vi "Get Index By Serial Number.vi"(8 "error in (no error)":errorcluster, 11 "Serial Number":string) -> (0 "error out":errorcluster, 3 "Index":i32)   [LabVIEW 2014]
doc: "Get device index by USB serial string descriptor."
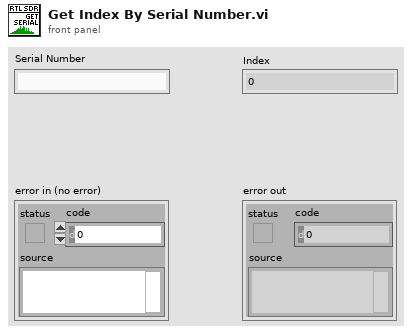
[diagram p1: front panel]
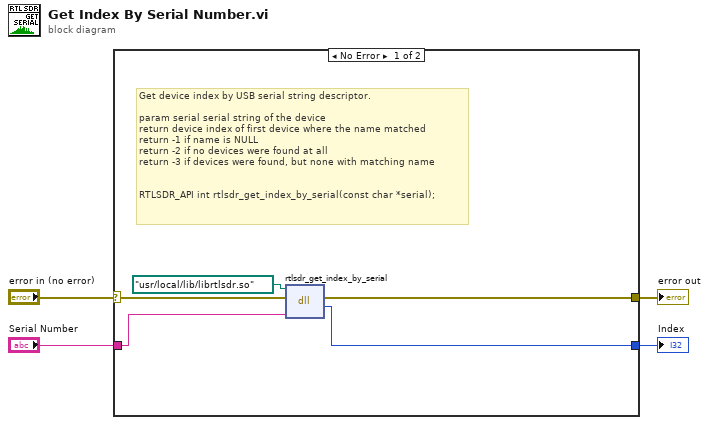
[diagram p0: block diagram]
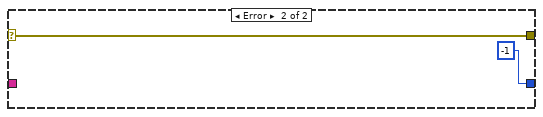
[diagram p2: hidden frame]
diagram:
  n1 = case shown="No Error" "error in (no error)" {
    selector: "error in (no error)" -> [w5 w11]
    tunnel: [w9 -1 ("return type")] -> w4
    tunnel: "Serial Number" -> [w8 _]
    tunnel: [w7 w11] -> w2
    frame No Error {
      # "Get device index by USB serial string descriptor.\n\nparam serial serial string of the device\nreturn device index of first device where the name matched\nreturn -1 if name is NULL\nreturn -2 if no devices were found at all\nreturn -3 if devices were found, but none with matching name\n\n\nRTLSDR_API int rtlsdr_get_index_by_serial(const char *serial);"
      n2 = dll-call lib="C:/Program Files (x86)/National Instruments/LabVIEW 2016/user.lib/rtlsdr/rtlsdr.*" fn="rtlsdr_get_index_by_serial"(path in=path "/usr/local/lib/librtlsdr.so", error in=w5, "serial"=w8) -> (error out=w7:errorcluster, "return type"=w9:i32)  [unwired: 2 in, 1 out]
    }
    frame Error {
    }
  }
  "Index" <- w4
  "error out" <- w2
